vi "Terminal.vi"(8 "error in":errorcluster) -> (0 "error out":errorcluster, 2 "ErrorOut":string, 3 "Output":string)   [LabVIEW 2017]
panel:
  in  "ProcessName":string="cmd"
  in  "Stop Button":bool
  in  "Input":string
  # "COMMAND PROMPT"
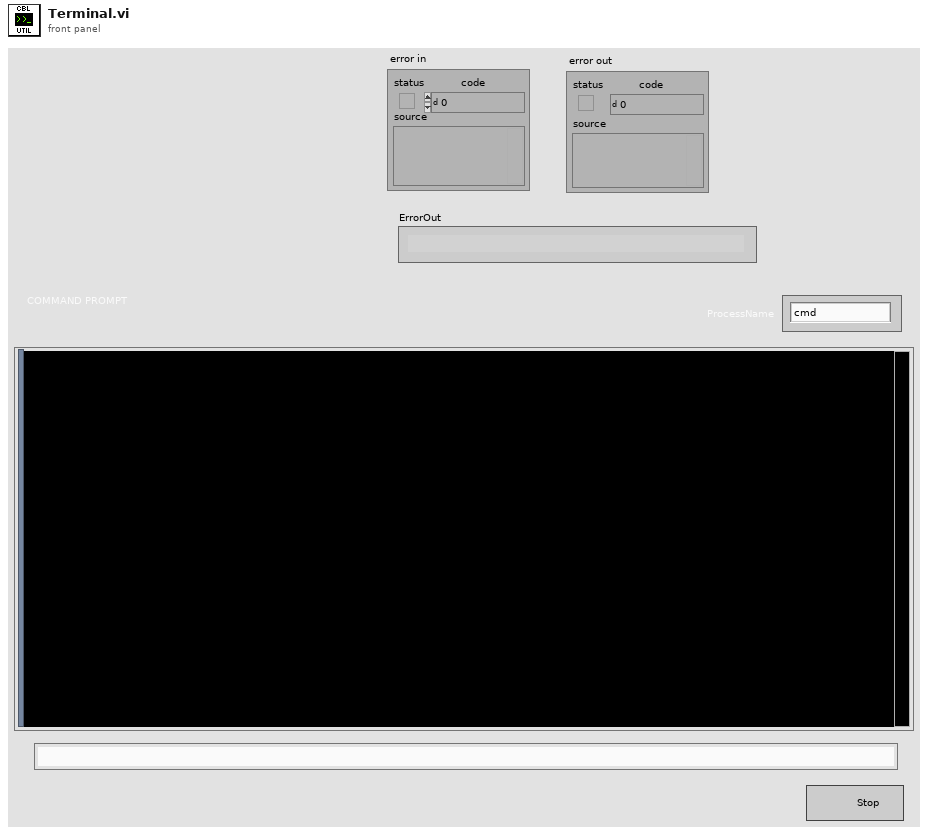
[diagram p1: front panel]
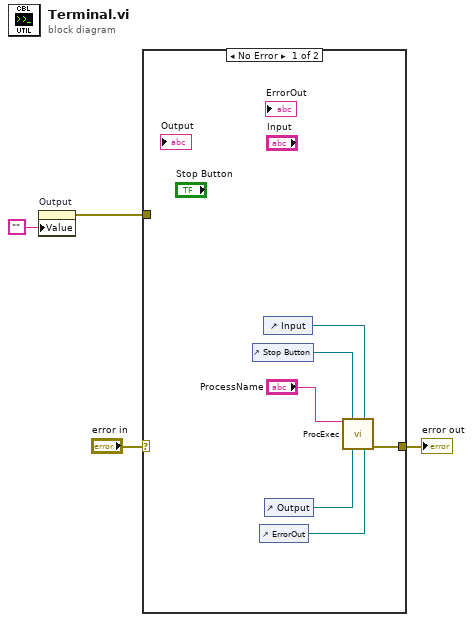
[diagram p0: block diagram]
diagram:
  n1 = property on="Output" class="Str"("Value"="") -> (error out=w2:errorcluster)  [unwired: 2 in, 1 out]
  n2 = case shown="No Error" "error in" {
    selector: "error in" -> [_ w11]
    tunnel: [w10 w11] -> w4
    tunnel: w2 -> [_ _]
    frame No Error {
      n3 = control-ref of="Stop Button"() -> (w7:refnum<vi>)
      n4 = control-ref of="ErrorOut"() -> (w8:refnum<vi>)
      n5 = control-ref of="Input"() -> (w6:refnum<vi>)
      n6 = control-ref of="Output"() -> (w9:refnum<vi>)
      n7 = call "ProcExec.vi"("ProcessName"="ProcessName", "Stop Button Ref"=w7, "StreamWrite String Ref"=w6, "StreamOut String Ref"=w9, "StreamErr String Ref"=w8) -> ("error out"=w10:errorcluster)  [unwired: 10 in]
    }
    frame Error {
    }
  }
  "error out" <- w4
